vi "Configure RF Channel.vi"(0 "VISA resource name":refnum<visa-resource-name>, 1 "RF Channel (0:Normal)":u16(ring) items=["Normal", "Average", "Amplitude", "Phase", "Frequency", "Maximum Peak Hold", "Minimum Peak Hold"], 2 "Averaging Sample Size (2)":i16=2 min=2 max=512 step=1, 3 "Spectrum Mode (0: Triggered)":u16(ring) items=["Triggered", "Free Run"], 4 "Start Frequency (0)":dbl min=0.0 step=0.1, 5 "error in (no error)":errorcluster, 6 "Enable RF Channel (T:Enable)":bool=TRUE, 7 "Start Units (0: Hz)":u16(ring) items=["Hz", "kHz", "MHz", "GHz"], 8 "Auto RF Detection (T:Enable)":bool=TRUE, 9 "Stop Frequency (0)":dbl min=0.0 step=0.1, 10 "Manual RF Detection (3: Average)":u16(ring)=3 items=["Positive Peak", "Negative Peak", "Sample", "Average"], 11 "Stop Units (2: MHz)":u16(ring)=2 items=["Hz", "kHz", "MHz", "GHz"]) -> (14 "VISA resource name out":refnum<visa-resource-name>, 19 "error out":errorcluster)   [LabVIEW 2016, in "Tektronix DPO MSO 2000 4000 Series.lvlib"]
doc: "Configures Spectrum Mode, Spectral Range, RF Detection and the various RF Channels for MDO series oscilloscopes.\n\n<B>Note:</B>\n This VI is applicable only to <B>MDO series</B> oscilloscopes."
uses:
  Tektronix DPO MSO 2000 4000 Series.lvlib
panel:
  # "RF Channel"
  # "RF Average"
  # "RF Spectrum"
  # "RF Detection Method"
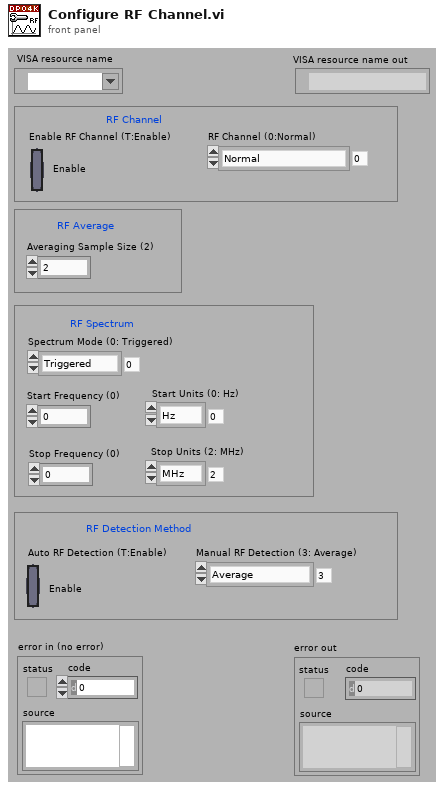
[diagram p1: front panel]
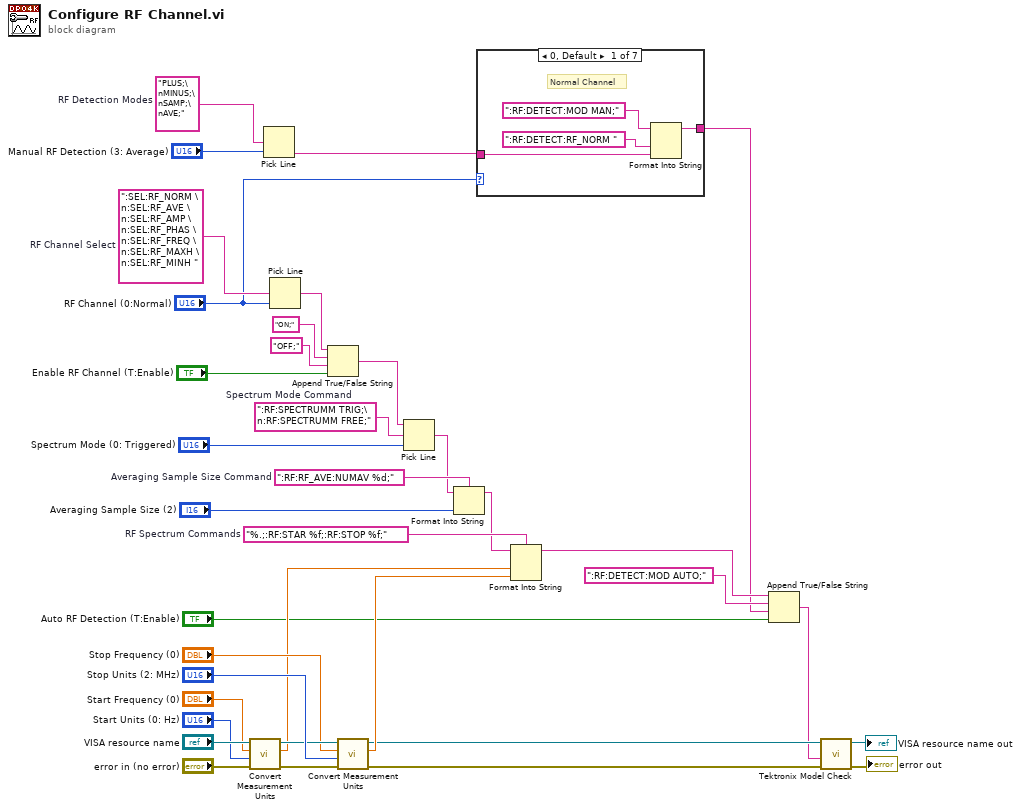
[diagram p0: block diagram]
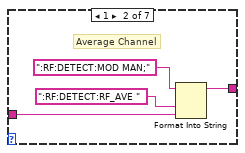
[diagram p2: hidden frame]
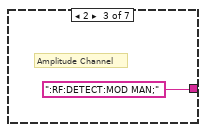
[diagram p3: hidden frame]
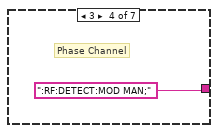
[diagram p4: hidden frame]
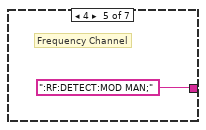
[diagram p5: hidden frame]
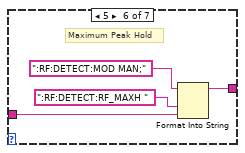
[diagram p6: hidden frame]
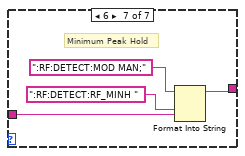
[diagram p7: hidden frame]
diagram:
  w11 = "PLUS;\nMINUS;\nSAMP;\nAVE;"  # RF Detection Modes
  w19 = ":RF:RF_AVE:NUMAV %d;"  # Averaging Sample Size Command
  w28 = "%.;:RF:STAR %f;:RF:STOP %f;"  # RF Spectrum Commands
  w29 = ":RF:SPECTRUMM TRIG;\n:RF:SPECTRUMM FREE;"  # Spectrum Mode Command
  w36 = ":SEL:RF_NORM \n:SEL:RF_AVE \n:SEL:RF_AMP \n:SEL:RF_PHAS \n:SEL:RF_FREQ \n:SEL:RF_MAXH \n:SEL:RF_MINH "  # RF Channel Select
  n1 = call "Convert Measurement Units.vi"("error in (no error)"="error in (no error)", "Units (0:Hz)"="Start Units (0: Hz)", "Measurement Value (0)"="Start Frequency (0)", "VISA resource name"="VISA resource name") -> ("error out"=w21:errorcluster, "Final Value"=w16:dbl, "VISA resource name out"=w22:refnum<visa-resource-name>)  [unwired: 5 in]
  n2 = Pick Line(multi-line string=w11, line index="Manual RF Detection (3: Average)") -> (output string=w10:string)  [unwired: 1 in]
  n3 = Pick Line(multi-line string=w36, line index="RF Channel (0:Normal)") -> (output string=w35:string)  [unwired: 1 in]
  n4 = Append True/False String(1:"Enable RF Channel (T:Enable)", 2:"OFF;" ("false string"), 3:"ON;" ("true string"), 4:w35) -> (0:w30:string)
  n5 = call "Convert Measurement Units.vi"("error in (no error)"=w21, "Units (0:Hz)"="Stop Units (2: MHz)", "Measurement Value (0)"="Stop Frequency (0)", "VISA resource name"=w22) -> ("error out"=w4:errorcluster, "Final Value"=w15:dbl, "VISA resource name out"=w5:refnum<visa-resource-name>)  [unwired: 5 in]
  n6 = Pick Line(string ("")=w30, multi-line string=w29, line index="Spectrum Mode (0: Triggered)") -> (output string=w18:string)
  n7 = Format Into String(format string=w19, initial string=w18, "Averaging Sample Size (2)") -> (resulting string=w14:string)  [unwired: 1 in, 1 out]
  n8 = case shown="0, Default" "RF Channel (0:Normal)" {
    tunnel: w10 -> [w39 w44 _ _ _ w50 w55]
    tunnel: [w38 w42 ":RF:DETECT:MOD MAN;" ("false string") ":RF:DETECT:MOD MAN;" ("false string") ":RF:DETECT:MOD MAN;" ("false string") w49 w53] -> w6
    frame 0, Default {
      # "Normal Channel"
      n9 = Format Into String(initial string=":RF:DETECT:MOD MAN;" ("false string"), ":RF:DETECT:RF_NORM " ("output string"), w39) -> (resulting string=w38:string)  [unwired: 2 in, 1 out]
    }
    frame 1 {
      # "Average Channel"
      n10 = Format Into String(initial string=":RF:DETECT:MOD MAN;" ("false string"), ":RF:DETECT:RF_AVE " ("output string"), w44) -> (resulting string=w42:string)  [unwired: 2 in, 1 out]
    }
    frame 2 {
      # "Amplitude Channel"
    }
    frame 3 {
      # "Phase Channel"
    }
    frame 4 {
      # "Frequency Channel"
    }
    frame 5 {
      # "Maximum Peak Hold"
      n11 = Format Into String(initial string=":RF:DETECT:MOD MAN;" ("false string"), ":RF:DETECT:RF_MAXH " ("output string"), w50) -> (resulting string=w49:string)  [unwired: 2 in, 1 out]
    }
    frame 6 {
      # "Minimum Peak Hold"
      n12 = Format Into String(initial string=":RF:DETECT:MOD MAN;" ("false string"), ":RF:DETECT:RF_MINH " ("output string"), w55) -> (resulting string=w53:string)  [unwired: 2 in, 1 out]
    }
  }
  n13 = Format Into String(format string=w28, initial string=w14, w16, w15) -> (resulting string=w8:string)  [unwired: 1 in, 1 out]
  n14 = Append True/False String(1:"Auto RF Detection (T:Enable)", 2:w6, 3:":RF:DETECT:MOD AUTO;" ("true string"), 4:w8) -> (0:w3:string)
  n15 = call "Tektronix Model Check.vi"("error in (no error)"=w4, "Command String"=w3, "VISA resource name"=w5) -> ("error out"=→"error out":errorcluster, "VISA resource name out"=→"VISA resource name out":refnum<visa-resource-name>)  [unwired: 7 in]
